vi "Run.vi"(8 "error in (no error)":errorcluster, 11 "App in":refnum<class "App.lvclass">) -> (0 "error out":errorcluster, 3 "App out":refnum<class "App.lvclass">)   [LabVIEW 2020, in "App.lvclass"]
uses:
  App.lvclass
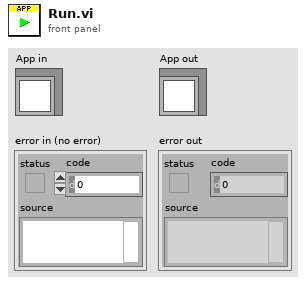
[diagram p1: front panel]
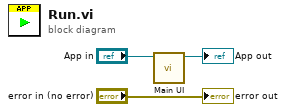
[diagram p0: block diagram]
diagram:
  n1 = call "Main UI.vi"("App in"="App in") -> ("App"=→"App out":refnum<class "App.lvclass">)  [unwired: 10 in]
  "error out" <- "error in (no error)"
